vi "ToString.vi"(8 "error in":errorcluster, 11 "String in":refnum<class "Generic.lvclass">) -> (0 "error out":errorcluster, 3 "String out":refnum<class "String.lvclass">)   [LabVIEW 2014, in "String.lvclass"]
uses:
  String.lvclass
  Generic/Generic.lvclass
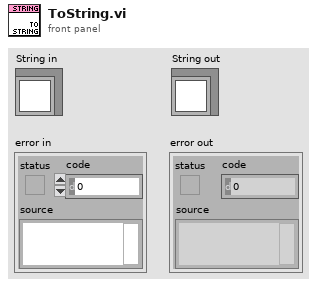
[diagram p1: front panel]
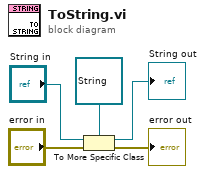
[diagram p0: block diagram]
diagram:
  n1 = To More Specific Class(target class=refnum<class "String.lvclass"> refnum ("String in"), reference="String in", error in="error in") -> (specific class reference=→"String out":refnum<class "String.lvclass">, error out=→"error out":errorcluster)
